vi "DFD Narrowband Filtering with State (Wfm).vi"(6 "state in":cluster{"state ":dbl[]}[](array[cluster]), 8 "error in (no error)":errorcluster, 10 "narrowband filter":T1 {"multirate filters"."mMRate_SumWl" min=1 max=32 step=1; "multirate filters"."mMRate_InputIwl" min=1 max=32 step=1; "multirate filters"."mMRate_GainWl" min=1 max=32 step=1; "multirate filters"."mMRate_OutputWl" min=1 max=32 step=1; "multirate filters"."mMRate_InputWl" min=1 max=32 step=1; "multirate filters"."mMRate_CoefWl" min=1 max=32 step=1; "multirate filters"."mMRate_Mode" items=["Default"=-1, "No Rate Change"=0, "Interpolation"=1, "Decimation"=2, "Interpolated"=3, "Rational"=4]}, 11 "signal in":waveform(dbl)={"t0"=timestamp(0 s since 1904-01-01), "dt"=0.0, "Y"=[]}) -> (0 "error out":errorcluster, 3 "signal out":waveform(dbl), 4 "state out":cluster{"state ":dbl[]}[](array[cluster]))   [LabVIEW 2017, in "NI_DigFilterLicensed.lvlib"]
doc: "Filters a signal with a narrowband filter. You must specify the initial internal states in <B>state in</B> to generate an accurate output. Wire data to the <B>signal in</B> input to determine the polymorphic instance to use or manually select the instance."
uses:
  <vilib>/addons/Digital Filter Design/NI_DigFilterLicensed.lvlib
  <vilib>/addons/Digital Filter Design/_Objects.llb/DFD Narrowband Filter Obj.ctl
  <vilib>/addons/Digital Filter Design/_Objects.llb/DFD Multirate Filter Obj.ctl
  <vilib>/addons/Digital Filter Design/_Objects.llb/DFD Multirate Mode.ctl
  <vilib>/addons/Digital Filter Design/_Objects.llb/DFD Coef Norm Type.ctl
  <vilib>/addons/Digital Filter Design/_Objects.llb/DFD Round-off Mode.ctl
  <vilib>/addons/Digital Filter Design/_Objects.llb/DFD FXP MRate Multiply Mode.ctl
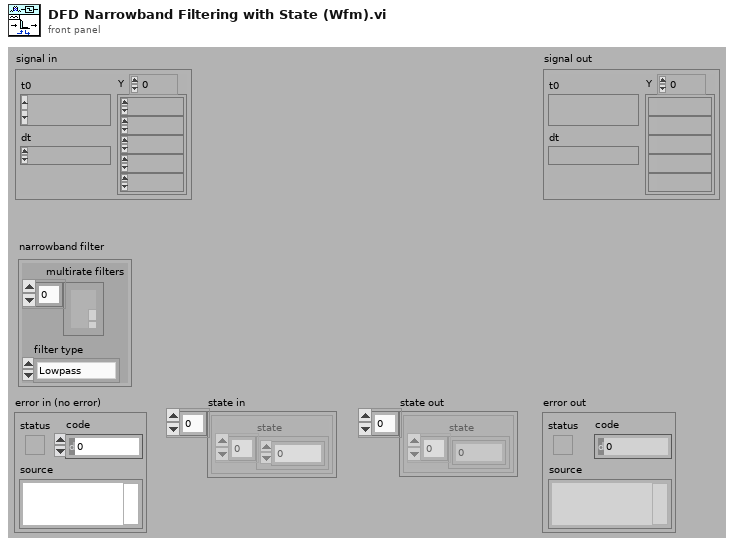
[diagram p1: front panel]
types:
  T1 = typedef "NI_DigFilterLicensed.lvlib/DFD Narrowband Filter Obj.ctl" = cluster{"multirate filters":T2[], "filter type":enum32{"Lowpass", "Highpass", "Bandpass", "Bandstop", "Wideband-Lowpass", "Wideband-Highpass"}}
  T2 = typedef "NI_DigFilterLicensed.lvlib/DFD Multirate Filter Obj.ctl" = cluster{"mMRate_Structure":enum16{"CIC", "FIR", "IIR", "Lattice"}, "mMRate_Mode":T3, "mMRate_Factor":i32, "mMRate_FIRParams":cluster{"mMRate_FIR_H":dbl[], "mMRate_FIR_IsNyquist?":bool, "mMRate_FIR_IsSymmetric?":bool}, "mMRate_CICParams":cluster{"mMRate_CIC_#Stage":i32, "mMRate_CIC_Lag":i32, "mMRate_CIC_Type":enum16{"Lowpass", "Highpass"}}, "mMRate_Order":i32, "mMRate_Version":string, "mMRate_Comments":string, "mMRate_RationalFactor":cluster{"mMRate_L":i32, "mMRate_M":i32}, "mMRate_Fs":dbl, "mMRate_Quantized?":bool, "mMRate_QFilterGain":dbl, "mMRate_CoefWl":i16, "mMRate_Scaling":cluster{"mMRate_ScaleByPowerOf2?":bool, "mMRate_ScaleType":T4}, "mMRate_InputWl":i16, "mMRate_OutputWl":i16, "mMRate_OutputMode":T5, "mMRate_MultMode":T6, "mMRate_BitPruning":bool, "mMRate_GainWl":i16, "mMRate_OutputFwl":i16, "mMRate_SumIwl":i16, "mMRate_InputIwl ":i16, "mMRate_SumWl":i16, "mMRate_CoefIwl":i16}
  T3 = typedef "NI_DigFilterLicensed.lvlib/DFD Multirate Mode.ctl" = i16
  T4 = typedef "NI_DigFilterLicensed.lvlib/DFD Coef Norm Type.ctl" = enum16{"No Norm", "Time Domain 1-Norm", "Time Domain 2-Norm", "Time Domain Inf-Norm"}
  T5 = typedef "NI_DigFilterLicensed.lvlib/DFD Round-off Mode.ctl" = enum16{"Nearest", "Truncation"}
  T6 = typedef "NI_DigFilterLicensed.lvlib/DFD FXP MRate Multiply Mode.ctl" = enum16{"Truncated", "Full"}
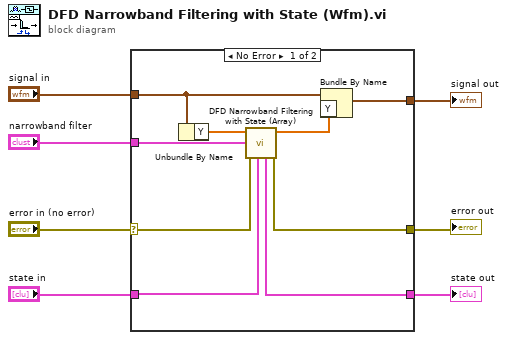
[diagram p0: block diagram]
diagram:
  n1 = case shown="No Error" "error in (no error)" {
    selector: "error in (no error)" -> [w9 w17]
    tunnel: [w8 w17] -> w6
    tunnel: "narrowband filter" -> [w11 _]
    tunnel: "signal in" -> [w10 _]
    tunnel: [w15 _] -> w4
    tunnel: [w14 _] -> w2
    tunnel: "state in" -> [w12 _]
    frame No Error {
      n2 = Unbundle By Name(w10) -> ("Y"=w13:dbl[])
      n3 = call <vilib>:"DFD Narrowband Filtering with State (Array).vi"("state in"=w12, "error in (no error)"=w9, "narrowband filter"=w11, "signal in"=w13) -> ("error out"=w8:errorcluster, "signal out"=w16:dbl[], "state out"=w14:cluster{"state ":dbl[]}[])  [unwired: 5 out]
      n4 = Bundle By Name(cluster=w10, "Y"=w16) -> (w15:waveform(dbl))
    }
    frame Error {
    }
  }
  "error out" <- w6
  "signal out" <- w4
  "state out" <- w2
